vi "Evaluate Expression.vi"(7 "expression":string) -> (8 "result":dbl format="%.2f", 15 "error out":errorcluster)   [LabVIEW 2012]
uses:
  subvis/private/LuaVIEW Push (string).vi
  subvis/private/LuaVIEW Pull (number).vi
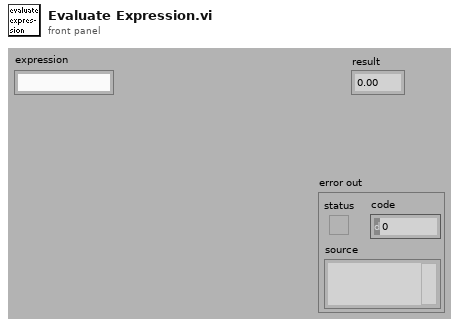
[diagram p1: front panel]
types:
  T1 = typedef "t_LuaVIEW Reference.ctl" = refnum<k1>
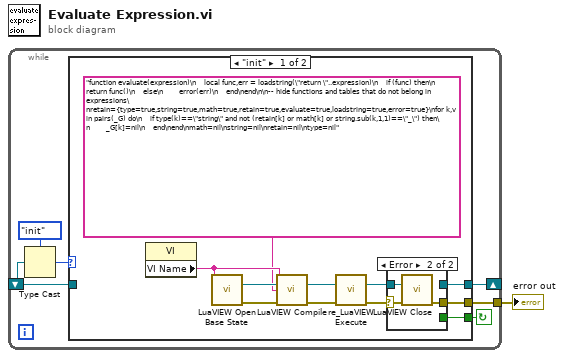
[diagram p0: block diagram]
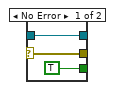
[diagram p2: hidden frame]
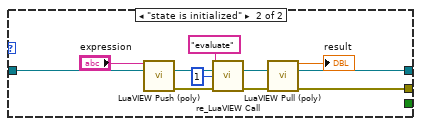
[diagram p3: hidden frame]
diagram:
  n1 = while {
    shift-right: [w7] -> _
    shift-left: _ -> [w6]
    tunnel: [w2] -> w1
    stop <- w3 continue-if-true
    n2 = Type Cast(type=enum32{"init", "state is initialized"}."init", x=w6) -> (*(type *) &x=w4:enum32{"init", "state is initialized"})
    n3 = case shown="\"init\"" w4 {
      tunnel: [w10 w34] -> w7
      tunnel: [w9 w25] -> w2
      tunnel: w6 -> [_ w35]
      tunnel: [w11 _] -> w3
      frame "init" {
        n4 = property class="VI"() -> ("VI Name"=w14:string)  [unwired: 2 in, 2 out]
        n5 = call "LuaVIEW Open Base State.vi"("close identifier (none)"=w14) -> ("LuaVIEW reference"=w16:T1, "error out"=w18:errorcluster)  [unwired: 13 in]
        n6 = call "LuaVIEW Compile.vi"("script name"=w14, "LuaVIEW reference in"=w16, "script"="function evaluate(expression)\n    local func,err = loadstring(\"return \"..expression)\n    if (func) then\n        return func()\n    else\n        error(err)\n    end\nend\n\n-- hide functions and tables that do not belong in expressions\nretain={type=true,string=true,math=true,retain=true,evaluate=true,loadstring=true,error=true}\nfor k,v in pairs(_G) do\n    if type(k)==\"string\" and not (retain[k] or math[k] or string.sub(k,1,1)==\"_\") then\n        _G[k]=nil\n    end\nend\nmath=nil\nstring=nil\nretain=nil\ntype=nil", "error in (no error)"=w18) -> ("LuaVIEW reference out"=w15:T1, "error out"=w17:errorcluster)  [unwired: 10 in]
        n7 = call "re_LuaVIEW Execute.vi"("LuaVIEW reference in"=w15, "error in (no error)"=w17) -> ("LuaVIEW reference out"=w12:T1, "error out"=w8:errorcluster)  [unwired: 12 in]
        n8 = case shown="Error" w8 {
          selector: w8 -> [w20 w24]
          tunnel: w12 -> [w21 w23]
          tunnel: [w20 w22] -> w9
          tunnel: [w21 _] -> w10
          tunnel: [TRUE _] -> w11
          frame No Error {
          }
          frame Error {
            n9 = call "LuaVIEW Close.vi"("LuaVIEW reference"=w23, "error in (no error)"=w24) -> ("dup error"=w22:errorcluster)  [unwired: 13 in]
          }
        }
      }
      frame "state is initialized" {
        n10 = call-poly "LuaVIEW Push (poly).vi"("string"="expression", "LuaVIEW reference in"=w35) -> ("LuaVIEW reference out"=w32:T1, "error out"=w33:errorcluster)  [unwired: 12 in]
        n11 = call "re_LuaVIEW Call.vi"("function name"="evaluate", "LuaVIEW reference in"=w32, "required results (no checking needed)"=1, "error in (no error)"=w33) -> ("LuaVIEW reference out"=w29:T1, "error out"=w30:errorcluster)  [unwired: 10 in]
        n12 = call-poly "LuaVIEW Pull (poly).vi"("LuaVIEW reference in"=w29, "error in (no error)"=w30) -> ("number"=→"result":dbl, "LuaVIEW reference out"=w34:T1, "error out"=w25:errorcluster)  [unwired: 11 in]
      }
    }
  }
  "error out" <- w1
